vi "20[2]-S7F23 Function.vi"(8 "error in (no error)":errorcluster, 10 "SECS-II Class":refnum<class "SECS-II Class.lvclass">, 11 "20-Process Program Downloading in":refnum<class "20-Process Program Downloading.lvclass">) -> (0 "error out":errorcluster, 2 "SECS-II Class Out":refnum<class "SECS-II Class.lvclass">, 3 "20-Process Program Downloading out":refnum<class "20-Process Program Downloading.lvclass">)   [LabVIEW 2020, in "SECS Scenarios.lvlib" / "20-Process Program Downloading.lvclass"]
uses:
  20-Process Program Downloading.lvclass
  D:/Dropbox/SECS/SECS_GEM v1.1.0/Com/SECS Scenarios/Scenarios Class/Scenarios Class.lvclass
  SECS Communication/SECS-II Class/SECS-II Class.lvclass
  SECS Communication/S7 Message Class/S7 Message Class.lvclass
  D:/Dropbox/SECS/SECS_GEM v1.1.0/Com/SECS Communication/SECS-II Class/SECS-II Class.lvclass
  Scenarios Class/Reply State.ctl
  Scenarios Class/Scenarios Class.lvclass/Scenarios Class.ctl
  SECS Communication/S7 Message Class/S7F27.ctl
  Scenarios Class/Write Reply State.vi
  Scenarios Class/Read HSMS Class.vi
  SECS Communication/HSMS Class/HSMS Class.lvclass
  Scenarios Class/Scenarios Class.lvclass
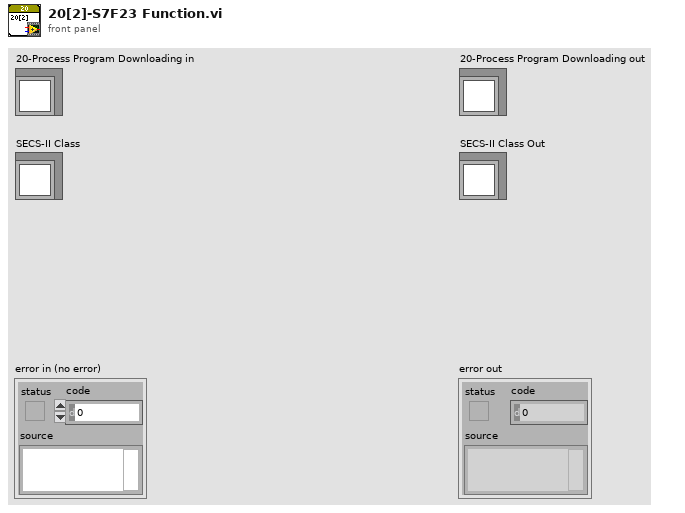
[diagram p1: front panel]
types:
  T1 = typedef "SECS Communication.lvlib/S7 Message Class.lvclass/S7F23.ctl" = cluster{"PPID":string, "MDLN":string, "SOFTREV":string, "Parameter":cluster{"CCODE":string, "PPARM":cluster{"Format Code":T2, "Value":variant}[]}[]}
  T2 = typedef "SECS Communication.lvlib/SECS-II Class.lvclass/Format Code.ctl" = enum16{"L", "A", "B", "Boolean", "J", "I1", "I2", "I4", "I8", "U1", "U2", "U4", "U8", "F4", "F8", "Char"}
  T3 = typedef "SECS Scenarios.lvlib/Scenarios Class.lvclass/Reply State.ctl" = enum16{"OK", "Illegal Data", "Unknown Stream", "Unknown Function", "Off-Line", "T3 Timeout", "Inner-Timeout"}
  T4 = typedef "SECS Communication.lvlib/S7 Message Class.lvclass/S7F27.ctl" = cluster{"PPID":string, "Verification":cluster{"ACKC7A":enum32{"ok", "inconsistent MDLN", "inconsistent SOFTREV", "invalid CCODE", "invalid PPARM value", "error described by ERRW7"}, "SEQNUM":u32, "ERRW7":string}[]}
  T5 = typedef "SECS Communication.lvlib/S7 Message Class.lvclass/S7F24.ctl" = enum8{"Accepted", "Permission not granted", "length error", "matrix overflow", "PPID not found", "unsupported mode", "initiated for asynchronous completion", "storage limit error"}
  T6 = cluster{"S7F24":T5, "Verification":cluster{"ACKC7A":enum32{"ok", "inconsistent MDLN", "inconsistent SOFTREV", "invalid CCODE", "invalid PPARM value", "error described by ERRW7"}, "SEQNUM":u32, "ERRW7":string}[]}
  T7 = cluster{"ACKC7A":enum32{"ok", "inconsistent MDLN", "inconsistent SOFTREV", "invalid CCODE", "invalid PPARM value", "error described by ERRW7"}, "SEQNUM":u32, "ERRW7":string}[]
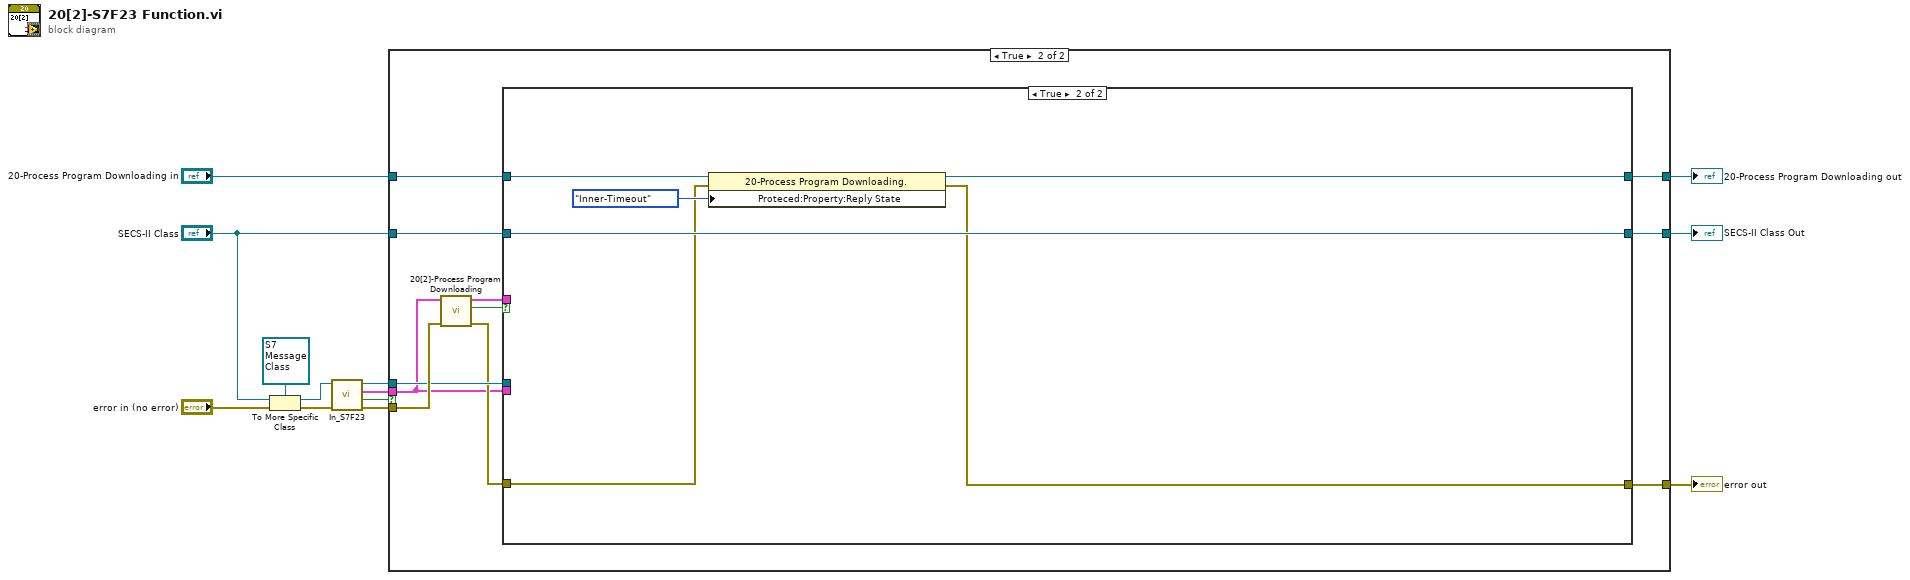
[diagram p0: block diagram]
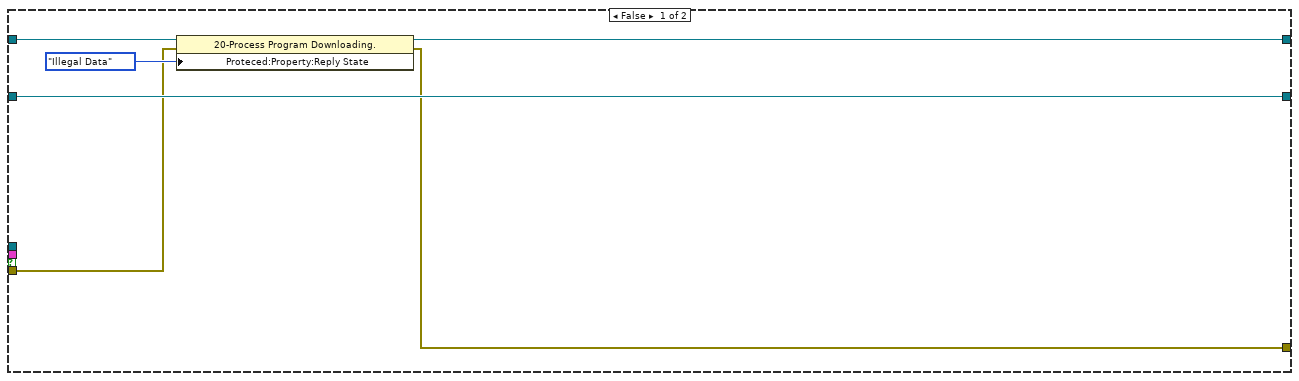
[diagram p2: hidden frame]
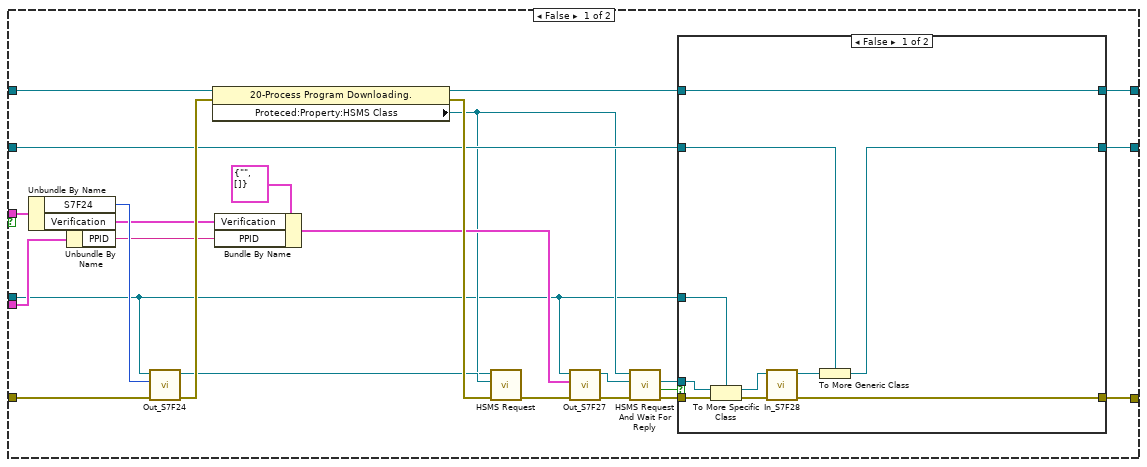
[diagram p3: hidden frame]
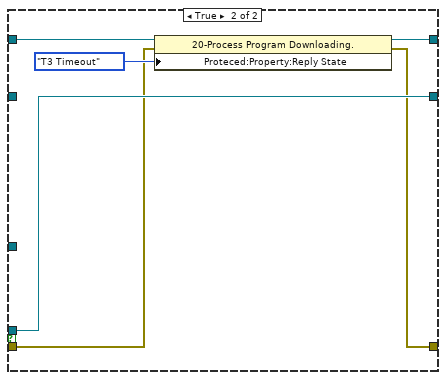
[diagram p4: hidden frame]
diagram:
  n1 = To More Specific Class(target class=refnum<class "S7 Message Class.lvclass"> refnum ("S7 Message Class in"), reference="SECS-II Class", error in="error in (no error)") -> (specific class reference=w11:refnum<class "S7 Message Class.lvclass">, error out=w12:errorcluster)
  n2 = call "In_S7F23.vi"("error in (no error)"=w12, "S7 Message Class in"=w11) -> ("error out"=w10:errorcluster, "OK?"=w1:bool, "S7F23"=w6:T1, "S7 Message Class out"=w9:refnum<class "S7 Message Class.lvclass">)  [unwired: 6 in]
  n3 = case shown="True" w1 {
    tunnel: w10 -> [w16 w30]
    tunnel: w9 -> [_ w29]
    tunnel: "20-Process Program Downloading in" -> [w18 w25]
    tunnel: w6 -> [_ w24]
    tunnel: [w15 w23] -> w5
    tunnel: [w14 w22] -> w4
    tunnel: "SECS-II Class" -> [w19 w21]
    tunnel: [w19 w20] -> w2
    frame False {
      n4 = property class="20-Process Program Downloading."(reference=w18, error in=w16, "Proteced:Property:Reply State"=Reply_State."Illegal Data" ("Reply State")) -> (reference out=w14:refnum<class "20-Process Program Downloading.lvclass">, error out=w15:errorcluster)
    }
    frame True {
      n5 = call "20[2]-Process Program Downloading.vi"("error in (no error)"=w30, "S7F23"=w24) -> ("error out"=w28:errorcluster, "Timeout?"=w26:bool, "Reply"=w27:T6)  [unwired: 7 in]
      n6 = case shown="True" w26 {
        tunnel: w25 -> [w55 w75]
        tunnel: w29 -> [w31 _]
        tunnel: [w37 w72] -> w23
        tunnel: [w35 w73] -> w22
        tunnel: w28 -> [w53 w74]
        tunnel: w27 -> [w51 _]
        tunnel: w24 -> [w46 _]
        tunnel: w21 -> [w34 w77]
        tunnel: [w32 w77] -> w20
        frame False {
          n7 = Unbundle By Name(w51) -> ("S7F24"=w50:T5, "Verification"=w44:T7)
          n8 = Unbundle By Name(w46) -> ("PPID"=w45:string)
          n9 = call "Out_S7F24.vi"("error in (no error)"=w53, "S7F24"=w50, "S7 Message Class in"=w31) -> ("error out"=w52:errorcluster, "S7 Message Class out"=w48:refnum<class "S7 Message Class.lvclass">)  [unwired: 7 in]
          n10 = property class="20-Process Program Downloading."(reference=w55, error in=w52) -> (reference out=w36:refnum<class "20-Process Program Downloading.lvclass">, error out=w54:errorcluster, "Proteced:Property:HSMS Class"=w33:refnum<class "HSMS Class.lvclass">)
          n11 = Bundle By Name(cluster=T4 {"PPID"="", "Verification"=[]} ("S7F27"), "Verification"=w44, "PPID"=w45) -> (w43:T4)
          n12 = call "HSMS Request.vi"("error in (no error)"=w54, "SECS-II Class In"=w48, "HSMS Class in"=w33) -> ("error out"=w49:errorcluster)  [unwired: 7 in, 1 out]
          n13 = call "Out_S7F27.vi"("error in (no error)"=w49, "S7F27"=w43, "S7 Message Class in"=w31) -> ("error out"=w38:errorcluster, "S7 Message Class out"=w39:refnum<class "S7 Message Class.lvclass">)  [unwired: 7 in]
          n14 = call "HSMS Request And Wait For Reply.vi"("error in (no error)"=w38, "SECS-II Class In"=w39, "HSMS Class in"=w33) -> ("error out"=w40:errorcluster, "Timeout?"=w42:bool, "SECS-II Class Out"=w41:refnum<class "SECS-II Class.lvclass">)  [unwired: 5 in, 1 out]
          n15 = case shown="False" w42 {
            tunnel: w41 -> [w64 w71]
            tunnel: w40 -> [w65 w67]
            tunnel: [w61 w66] -> w37
            tunnel: w36 -> [w60 w70]
            tunnel: [w60 w69] -> w35
            tunnel: w34 -> [w57 _]
            tunnel: [w56 w71] -> w32
            tunnel: w31 -> [w59 _]
            frame False {
              n16 = To More Specific Class(target class=w59, reference=w64, error in=w65) -> (specific class reference=w62:refnum<class "S7 Message Class.lvclass">, error out=w63:errorcluster)
              n17 = call "In_S7F28.vi"("error in (no error)"=w63, "S7 Message Class in"=w62) -> ("error out"=w61:errorcluster, "S7 Message Class out"=w58:refnum<class "S7 Message Class.lvclass">)  [unwired: 7 in, 1 out]
              n18 = To More Generic Class(target class=w57, reference=w58) -> (generic class reference=w56:refnum<class "SECS-II Class.lvclass">)
            }
            frame True {
              n19 = property class="20-Process Program Downloading."(reference=w70, error in=w67, "Proteced:Property:Reply State"=Reply_State."T3 Timeout" ("Reply State")) -> (reference out=w69:refnum<class "20-Process Program Downloading.lvclass">, error out=w66:errorcluster)
            }
          }
        }
        frame True {
          n20 = property class="20-Process Program Downloading."(reference=w75, error in=w74, "Proteced:Property:Reply State"=Reply_State."Inner-Timeout" ("Reply State")) -> (reference out=w73:refnum<class "20-Process Program Downloading.lvclass">, error out=w72:errorcluster)
        }
      }
    }
  }
  "error out" <- w5
  "20-Process Program Downloading out" <- w4
  "SECS-II Class Out" <- w2
